vi "Set Average.vi"(8 "error in (no error)":errorcluster, 9 "firmware revision":string(combo), 10 "average (4)":i32=4 min=0 max=15, 11 "VISA resource name":refnum<visa-resource-name>) -> (0 "error out":errorcluster, 2 "bridge error":T1, 3 "VISA resource name out":refnum<visa-resource-name>)   [LabVIEW 2024, in "Andeen-Hagerling 2700A.lvlib"]
doc: "Sets the approximate time used to make a measurement."
uses:
  Andeen-Hagerling 2700A.lvlib
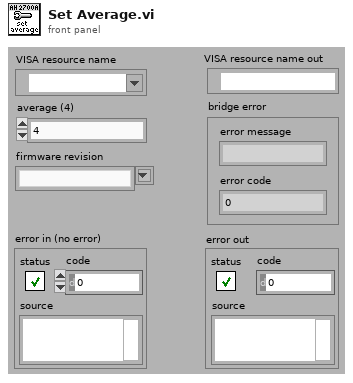
[diagram p1: front panel]
types:
  T1 = cluster{"error message":string, "error code":i32}
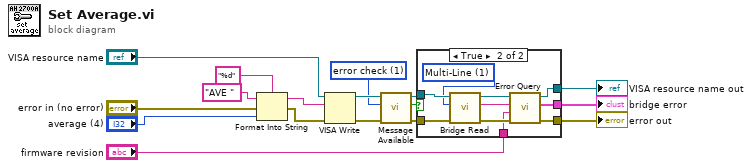
[diagram p0: block diagram]
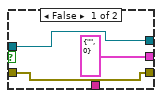
[diagram p2: hidden frame]
diagram:
  w1 = u16 1 items=["none", "error check", "multiline read", "infinite"] ("delay")
  n1 = Format Into String(format string="%d", initial string="AVE " ("command"), error in="error in (no error)", "average (4)") -> (resulting string=w13:string, error out=w14:errorcluster)
  n2 = VISA Write(VISA resource name="VISA resource name", write buffer=w13, error in (no error)=w14) -> (VISA resource name out=w10:refnum<visa-resource-name>, error out=w9:errorcluster)  [unwired: 1 out]
  n3 = call "Message Available.vi"("error in (no error)"=w9, "delay"=w1, "VISA resource name"=w10) -> ("error out"=w6:errorcluster, "message available"=w8:bool, "VISA resource name out"=w7:refnum<visa-resource-name>)  [unwired: 6 in]
  n4 = case shown="True" w8 {
    tunnel: w7 -> [w19 w27]
    tunnel: w6 -> [w20 w26]
    tunnel: "firmware revision" -> [_ w25]
    tunnel: [w20 w24] -> w4
    tunnel: [w19 w23] -> w3
    tunnel: [T1 {"error message"="", "error code"=0} ("bridge error") w22] -> w2
    frame False {
    }
    frame True {
      w21 = u16 1 items=["Single Line", "Multi-Line"] ("Multiline")
      n5 = call "Bridge Read.vi"("error in (no error)"=w26, "multiline"=w21, "VISA resource name"=w27) -> ("error out"=w29:errorcluster, "read buffer"=w30:string, "VISA resource name out"=w28:refnum<visa-resource-name>)  [unwired: 6 in]
      n6 = call "Error Query.vi"("error in (no error)"=w29, "firmware revision"=w25, "measurement line"=w30, "VISA resource name"=w28) -> ("error out"=w24:errorcluster, "bridge error"=w22:T1, "VISA resource name out"=w23:refnum<visa-resource-name>)  [unwired: 5 in]
    }
  }
  "VISA resource name out" <- w3
  "error out" <- w4
  "bridge error" <- w2
